vi "Record Nested Actor.vi"(8 "error in (no error)":errorcluster, 10 "Message Enqueuer":refnum<class "Message Enqueuer.lvclass">, 11 "Actor in":refnum<class "Actor.lvclass">) -> (3 "Actor out":refnum<class "Actor.lvclass">)   [LabVIEW 2020, in "Actor Framework.lvlib" / "Actor.lvclass"]
uses:
  <vilib>/ActorFramework/Actor/Actor.lvclass
  <vilib>/ActorFramework/Message Enqueuer/Message Enqueuer.lvclass
  <vilib>/ActorFramework/Actor/Actor.lvclass/Actor.ctl
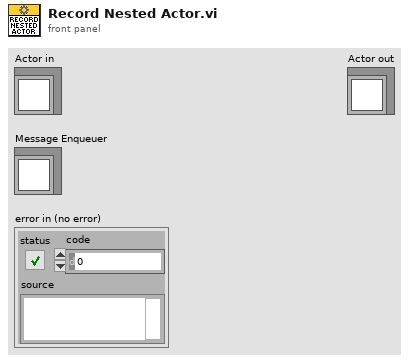
[diagram p1: front panel]
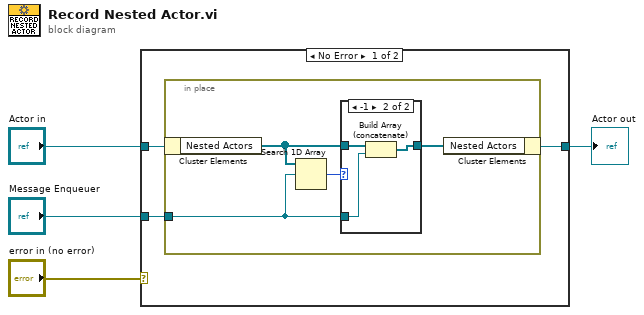
[diagram p0: block diagram]
diagram:
  n1 = case shown="No Error" "error in (no error)" {
    tunnel: [w6 w16] -> w3
    tunnel: "Actor in" -> [w7 w16]
    tunnel: "Message Enqueuer" -> [w5 _]
    frame No Error {
      n2 = in-place {
        in-place-border: w5 -> [w9]
        n3 = in-place-cluster #1(w7) -> ("Nested Actors"=w10:refnum<class "Message Enqueuer.lvclass">[])
        n4 = Search 1D Array(1D array=w10, element=w9) -> (index of element=w11:i32)  [unwired: 1 in]
        n5 = case shown="-1" w11 {
          tunnel: w10 -> [w12 w15]
          tunnel: w9 -> [_ w14]
          tunnel: [w12 w13] -> w8
          frame Default {
          }
          frame -1 {
            n6 = Build Array (concatenate)(w15, w14) -> (w13:refnum<class "Message Enqueuer.lvclass">[])
          }
        }
        n7 = in-place-cluster #1("Nested Actors"=w8) -> (w6:refnum<class "Actor.lvclass">)
      }
    }
    frame Error {
    }
  }
  "Actor out" <- w3
